vi "GetCursorPos.vi"(8 "error in (no error)":errorcluster) -> (0 "error out":errorcluster, 2 "Return":u32, 3 "lpPoint":cluster{"Numeric":i32, "Numeric":i32})   [LabVIEW 2019]
uses:
  user32.dll
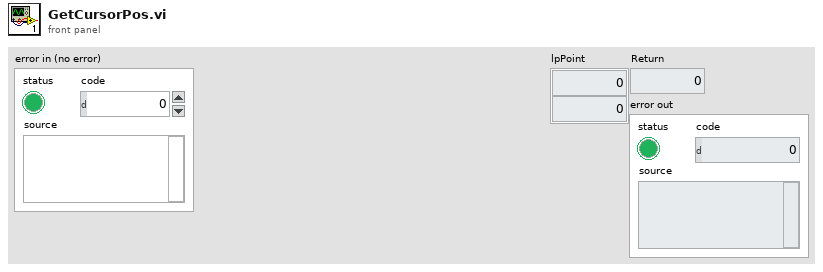
[diagram p1: front panel]
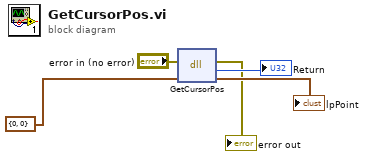
[diagram p0: block diagram]
diagram:
  n1 = dll-call lib="user32.dll" fn="GetCursorPos"(error in="error in (no error)", "lpPoint"=cluster{i32, i32} {0, 0}) -> (error out=→"error out":errorcluster, "Return"=→"Return":u32, "lpPoint"=→"lpPoint":cluster{i32, i32})  [unwired: 2 in, 1 out]
